vi "Insertion Tests.vi"() -> ()   [LabVIEW 2017]
uses:
  String Subset.vi
  Parsing/Parse Full Path or Item Name.vi
  Next JSON Value.vi
  support/Error Cluster From Code.vi
  Offset/Find Item Locations by Path.vi
  JSONtext.lvlib
  <vilib>/addons/_JKI Toolkits/Caraya/classes/Assert/Assert.lvclass
  <vilib>/addons/_JKI Toolkits/Caraya/classes/Test/Test.lvclass
panel:
  out "Found":bool
  out "Replaced if Found":bool
  out "<JSON>":string
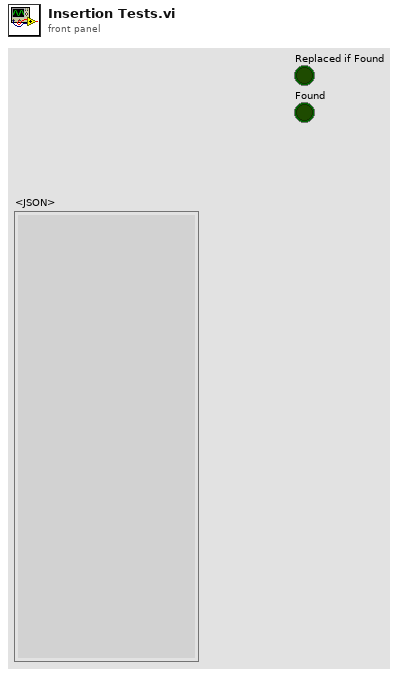
[diagram p1: front panel]
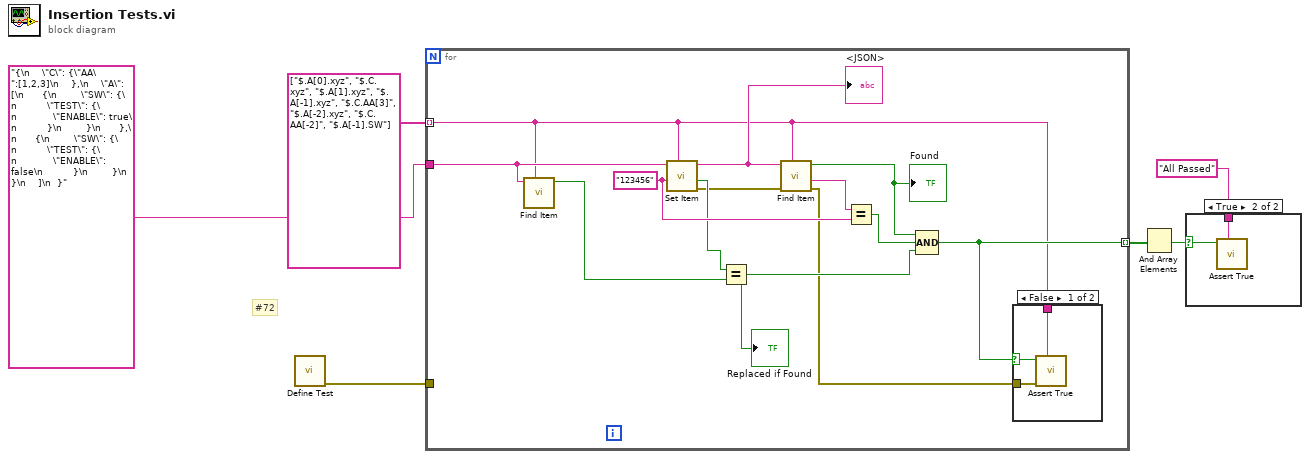
[diagram p0: block diagram]
diagram:
  # "#72"
  n1 = call <vilib>:"Define Test.vi"() -> ("error out"=w5:errorcluster)  [unwired: 11 in]
  n2 = for {
    tunnel: "{\n    \"C\": {\"AA\":[1,2,3]\n    },\n    \"A\": [\n      {\n        \"SW\": {\n          \"TEST\": {\n            \"ENABLE\": true\n          }\n        }\n      },\n      {\n        \"SW\": {\n          \"TEST\": {\n            \"ENABLE\": false\n          }\n        }\n      }\n    ]\n  }" -> [w13]
    tunnel: w5 -> [_]
    tunnel: string[] ["$.A[0].xyz", "$.C.xyz", "$.A[1].xyz", "$.A[-1].xyz", "$.C.AA[3]", "$.A[-2].xyz", "$.C.AA[-2]", "$.A[-1].SW"] -> [w12] mode=indexing
    tunnel: [w15] -> w3 mode=indexing
    w18 = "123456" ("JSON to Insert")
    n3 = call "Find Item.vi"("$Path or Item Name"=w12, "JSON"=w13) -> ("Found"=w10:bool)  [unwired: 6 in, 3 out]
    n4 = call "Set Item.vi"("$Path or Item Name"=w12, "JSON to Insert"=w18, "JSON"=w13) -> ("error out"=w8:errorcluster, "Replaced"=w11:bool, "<JSON>"=w14:string)  [unwired: 5 in]
    "<JSON>" <- w14
    n5 = Equal?(x=w11, y=w10) -> (x = y?=w9:bool)
    "Replaced if Found" <- w9
    n6 = call "Find Item.vi"("$Path or Item Name"=w12, "error in (no error)"=w8, "JSON"=w14) -> ("error out"=w7:errorcluster, "<JSON>"=w19:string, "Found"=w17:bool)  [unwired: 5 in, 1 out]
    "Found" <- w17
    n7 = Equal?(x=w19, y=w18) -> (x = y?=w16:bool)
    n8 = Compound Arithmetic op=AND(w17, w16, w9) -> (w15:bool)
    n9 = case shown="False" w15 {
      selector: w15 -> [w21 _]
      tunnel: w7 -> [w22 _]
      tunnel: w12 -> [w20 _]
      frame False {
        n10 = call <vilib>:"Assert True.vi"("Label"=w20, "error in (no error)"=w22, "True?"=w21) -> ()  [unwired: 8 in, 1 out]
      }
      frame True {
      }
    }
  }
  n11 = And Array Elements(Boolean array=w3) -> (logical AND=w2:bool)
  n12 = case shown="True" w2 {
    selector: w2 -> [_ w24]
    tunnel: "All Passed" -> [_ w23]
    frame False {
    }
    frame True {
      n13 = call <vilib>:"Assert True.vi"("Label"=w23, "True?"=w24) -> ()  [unwired: 9 in, 1 out]
    }
  }
